vi "LDR.vi"() -> ()   [LabVIEW 2020]
uses:
  <vilib>/MakerHub/LINX/Public/Peripherals/Analog/Analog Read 1 Chan.vi
  <vilib>/MakerHub/LINX/Public/Peripherals/Digital/Digital Write 1 Chan.vi
  <vilib>/MakerHub/LINX/Public/Peripherals/Analog/Analog Read N Chans.vi
  <vilib>/MakerHub/LINX/Public/Peripherals/Digital/Digital Write N Chans.vi
  <vilib>/MakerHub/LINX/Private/Local IO/LinxAnalogRead.vi
  <vilib>/MakerHub/LINX/Public/Utilities/Check Channel.vi
  <vilib>/MakerHub/LINX/Private/Local IO/LinxDigitalWrite.vi
  <vilib>/MakerHub/LINX/Public/Utilities/Open Serial.vi
  <vilib>/MakerHub/LINX/Private/Utilties/Generate Error.vi
  <vilib>/MakerHub/LINX/LMH-LINX.lvlib
panel:
  in  "Tab Control":T1(tab)
  in  "PORT CONFIGURATION":refnum<visa-resource-name>="N/A"
  in  "INPUT ANALOG PIN":dbl
  in  "INPUT DIGITAL PIN":dbl
  out "ELECTRICAL VOLTAGE":dbl(graph)
  out "LAMP CONDITION":bool
  in  "TURN  OFF   SYSTEM":bool
  out "VOLTAGE":dbl format="%_3g"
  out "SENSOR  GYRO":dbl
  out "SENSOR DHT11":dbl
  out "SENSOR PIR":dbl
  out "SENSOR LM35":dbl
  out "SENSOR  ULTRA":dbl
  out "SENSOR  POTENSIO":dbl
  out "SENSOR  LED":dbl
  out "SENSOR  LDR":dbl
  out "SENSOR  SUHU":dbl
  out "SENSOR AIR":dbl
  out "SENSOR  UDARA":dbl
  out "SENSOR  API":dbl
  out "SENSOR GETARAN":dbl
  out "SENSOR  ANGIN":dbl
  out "SENSOR  UAP":dbl
  out "SENSOR  GAS":dbl
  in  "SENSOR  GYRO":dbl
  in  "SENSOR DHT11":dbl
  in  "SENSOR PIR":dbl
  in  "SENSOR LM35":dbl
  in  "SENSOR  ULTRA":dbl
  in  "SENSOR  POTENSIO":dbl
  in  "SENSOR  LED":dbl
  in  "SENSOR  LDR":dbl
  in  "SENSOR  SUHU":dbl
  in  "SENSOR AIR":dbl
  in  "SENSOR  UDARA":dbl
  in  "SENSOR  API":dbl
  in  "SENSOR GETARAN":dbl
  in  "SENSOR  ANGIN":dbl
  in  "SENSOR  UAP":dbl
  in  "SENSOR  GAS":dbl
  # "WAREHOUSE INVENTORY SYSTEM MANAGEMENT"
  # "Selamat datang di Sistem Inventaris Gudang kami, yang dilengkapi sensor lampu LDR untuk pengawasan stok lebih aman dan efisien. Dengan sistem ini, pencatatan persediaan menjadi lebih mudah dan teratur, mendukung operasional gudang yang optimal. Selamat menggunakan!"
  # "RIZKI TRIAMADEWA\n223443069\n2AEC3"
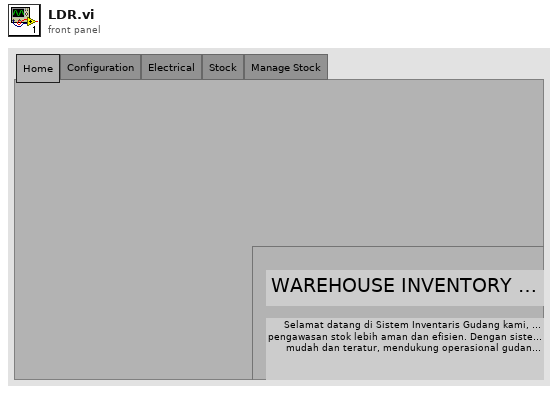
[diagram p1: front panel]
types:
  T1 = enum32{"Home", "Configuration", "Electrical", "Stock", "Manage Stock"}
  T2 = typedef "LMH-LINX.lvlib/LINX Ref.ctl" = cluster{"IO":T3, "Interface":T4, "LINX Device Config":T5}
  T3 = typedef "LMH-LINX.lvlib/Platform.ctl" = enum16{"Remote", "Local"}
  T4 = typedef "LMH-LINX.lvlib/Interface.ctl" = enum16{"Serial", "TCP"}
  T5 = typedef "LMH-LINX.lvlib/Device.lvlib/LINX Device Config.ctl" = cluster{"Interface":T4, "COM Port":refnum<visa-resource-name>, "TCP Configuration":T6, "Device Family":u8, "Device ID":u8, "Device Name":string, "TCP Ref":refnum<k5>, "Channels":T7}
  T6 = typedef "LMH-LINX.lvlib/Device.lvlib/TCP Config.ctl" = cluster{"IP Address":string, "Port":u16}
  T7 = typedef "LMH-LINX.lvlib/Channels.ctl" = cluster{"DI":u8[], "DO":u8[], "AI":u8[], "AO":u8[], "PWM":u8[], "QE":u8[], "UART":u8[], "I2C 2":u8[], "SPI":u8[], "CAN":u8[], "Servo":u8[], "AI Ref (V)":dbl, "AI Resolution (Bits)":u8, "AO Ref (V)":dbl, "AO Resolution (Bits)":u8}
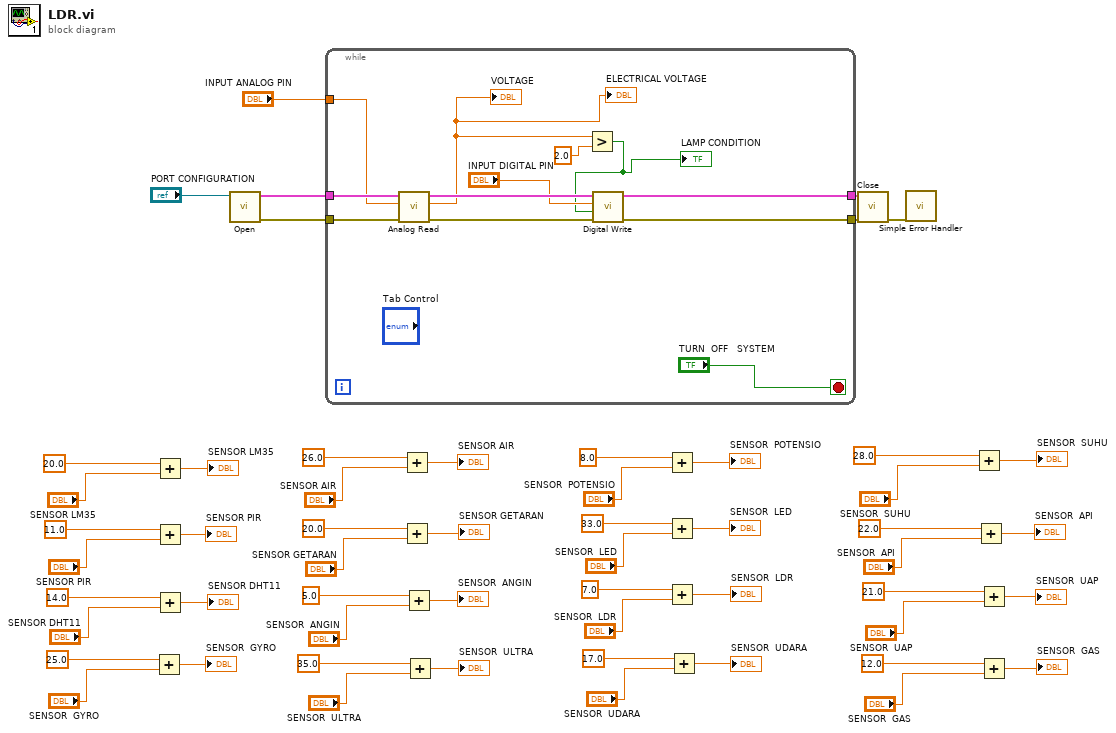
[diagram p0: block diagram]
diagram:
  n1 = Add(x=25.0 ("SENSOR  GYRO"), y="SENSOR  GYRO") -> (x+y=→"SENSOR  GYRO":dbl)
  n2 = Add(x=20.0 ("VOLTAGE 2"), y="SENSOR LM35") -> (x+y=→"SENSOR LM35":dbl)
  n3 = Add(x=11.0 ("SENSOR PIR"), y="SENSOR PIR") -> (x+y=→"SENSOR PIR":dbl)
  n4 = Add(x=14.0 ("SENSOR DHT11"), y="SENSOR DHT11") -> (x+y=→"SENSOR DHT11":dbl)
  n5 = call-poly <vilib>:"Open.vi"("Serial Port"="PORT CONFIGURATION") -> ("Error Out"=w53:errorcluster, "LINX Resource"=w54:T2)  [unwired: 8 in, 1 out]
  n6 = while {
    tunnel: w54 -> [w67]
    tunnel: w53 -> [w66]
    tunnel: [w63] -> w52
    tunnel: [w62] -> w51
    tunnel: "INPUT ANALOG PIN" -> [w61]
    stop <- "TURN  OFF   SYSTEM" stop-if-true
    n7 = call-poly <vilib>:"Analog Read.vi"("Error In"=w66, "Analog Channel"=w61, "LINX Resource"=w67) -> ("Error Out"=w64:errorcluster, "Voltage"=w56:dbl, "LINX Resource"=w65:T2)  [unwired: 5 in, 1 out]
    "ELECTRICAL VOLTAGE" <- w56
    "VOLTAGE" <- w56
    n8 = Greater?(x=w56, y=2.0) -> (0:w58:bool)
    "LAMP CONDITION" <- w58
    n9 = call-poly <vilib>:"Digital Write.vi"("Error In"=w64, "Output Value"=w58, "DO Channel"="INPUT DIGITAL PIN", "LINX Resource"=w65) -> ("Error Out"=w62:errorcluster, "LINX Resource"=w63:T2)  [unwired: 6 in]
  }
  n10 = Add(x=26.0 ("SENSOR AIR"), y="SENSOR AIR") -> (x+y=→"SENSOR AIR":dbl)
  n11 = Add(x=20.0 ("SENSOR GETARAN"), y="SENSOR GETARAN") -> (x+y=→"SENSOR GETARAN":dbl)
  n12 = Add(x=5.0 ("SENSOR  ANGIN"), y="SENSOR  ANGIN") -> (x+y=→"SENSOR  ANGIN":dbl)
  n13 = Add(x=35.0 ("SENSOR  ULTRA"), y="SENSOR  ULTRA") -> (x+y=→"SENSOR  ULTRA":dbl)
  n14 = Add(x=8.0 ("SENSOR  POTENSIO"), y="SENSOR  POTENSIO") -> (x+y=→"SENSOR  POTENSIO":dbl)
  n15 = Add(x=33.0 ("SENSOR  LED"), y="SENSOR  LED") -> (x+y=→"SENSOR  LED":dbl)
  n16 = Add(x=7.0 ("SENSOR  LDR"), y="SENSOR  LDR") -> (x+y=→"SENSOR  LDR":dbl)
  n17 = Add(x=17.0 ("SENSOR  UDARA"), y="SENSOR  UDARA") -> (x+y=→"SENSOR  UDARA":dbl)
  n18 = call <vilib>:"Close.vi"("Error In"=w51, "LINX Resource"=w52) -> ("Error Out"=w50:errorcluster)  [unwired: 9 in]
  n19 = call <vilib>:"Simple Error Handler.vi"("error in (no error)"=w50) -> ()  [unwired: 4 in, 5 out]
  n20 = Add(x=28.0 ("SENSOR  SUHU"), y="SENSOR  SUHU") -> (x+y=→"SENSOR  SUHU":dbl)
  n21 = Add(x=22.0 ("SENSOR  API"), y="SENSOR  API") -> (x+y=→"SENSOR  API":dbl)
  n22 = Add(x=21.0 ("SENSOR  UAP"), y="SENSOR  UAP") -> (x+y=→"SENSOR  UAP":dbl)
  n23 = Add(x=12.0 ("SENSOR  GAS"), y="SENSOR  GAS") -> (x+y=→"SENSOR  GAS":dbl)
